vi "DT3120_CloseDevice.vi"(8 "error in (no error)":errorcluster, 11 "lpDevId":i32) -> (0 "error out":errorcluster)   [LabVIEW 2010]
uses:
  olimg32.dll
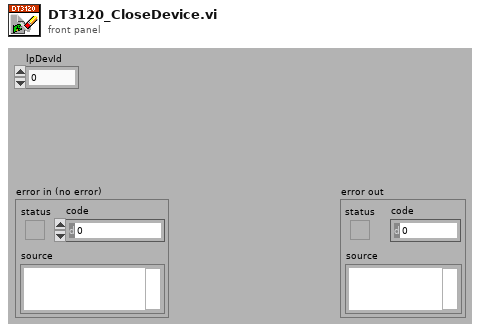
[diagram p1: front panel]
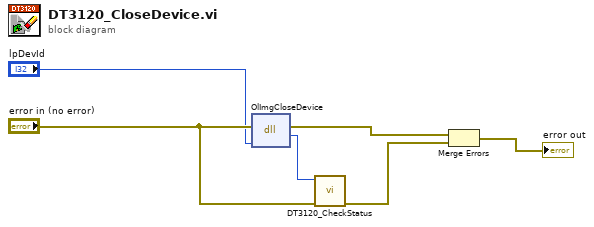
[diagram p0: block diagram]
diagram:
  n1 = dll-call lib="C:/LabVIEW Programs/MT Scan/SubVIs/olimg32.dll" fn="OlImgCloseDevice"(error in="error in (no error)", "DevId"="lpDevId") -> (error out=w4:errorcluster, "Status"=w6:u32)  [unwired: 3 in, 1 out]
  n2 = call "DT3120_CheckStatus.vi"("error in"="error in (no error)", "Status"=w6) -> ("error out"=w3:errorcluster)  [unwired: 9 out]
  n3 = Merge Errors(w4, w3) -> (→"error out":errorcluster)
